vi "Find Endpoint Configuration Section.vi"(8 "error in (no error)":errorcluster, 11 "SLSC Custom Device Ref in":T1 format="%.0x") -> (0 "error out":errorcluster, 2 "Endpoint Config Section Ref":T1 format="%.0x", 3 "SLSC Custom Device  Ref out":T1 format="%.0x")   [LabVIEW 2017, in "SLSC Switch Scripting.lvlib"]
uses:
  SLSC Switch Scripting.lvlib
  <vilib>/NI Veristand/Custom Device API/Custom Device Item Ref.ctl
  NationalInstruments.VeriStand.SystemDefinitionAPI
  SLSC Scripting Constants.vi
  <vilib>/NI VeriStand/Custom Device API/Custom Device API.lvlib
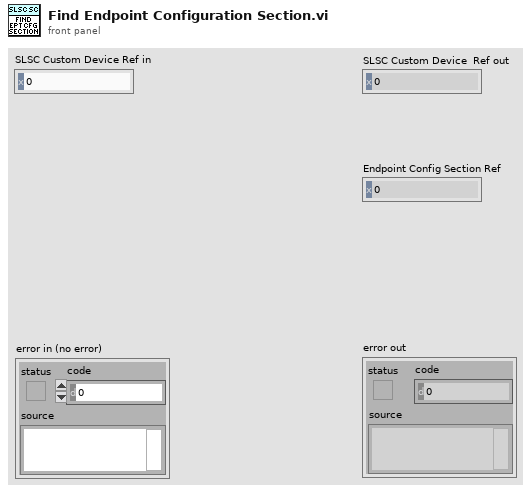
[diagram p1: front panel]
types:
  T1 = typedef "Custom Device API.lvlib/Custom Device Item Ref.ctl" = u64
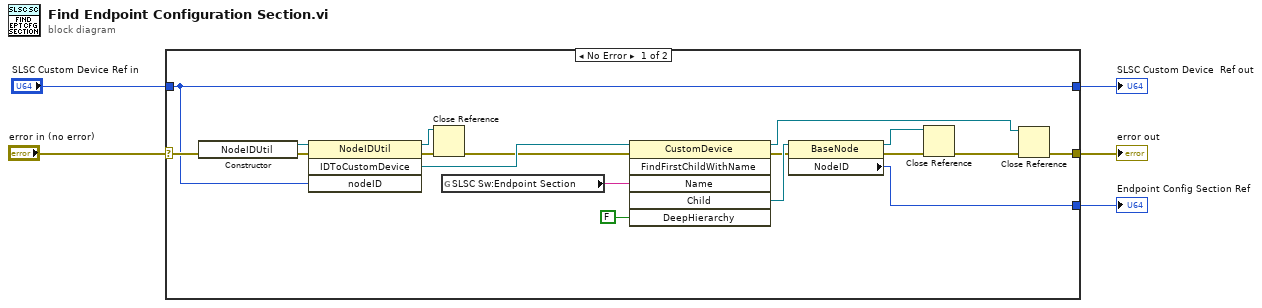
[diagram p0: block diagram]
diagram:
  n1 = case shown="No Error" "error in (no error)" {
    selector: "error in (no error)" -> [w15 w25]
    tunnel: "SLSC Custom Device Ref in" -> [w6 w24]
    tunnel: [w6 w24] -> w4
    tunnel: [w7 w25] -> w3
    tunnel: [w19 _] -> w1
    frame No Error {
      n2 = constructor class="NodeIDUtil"(error in=w15) -> (reference out=w17:refnum<k24>, error out=w18:errorcluster)  [unwired: 2 in, 1 out]
      n3 = invoke class="NodeIDUtil" method="IDToCustomDevice"(reference=w17, error in=w18, "nodeID"=w6) -> (reference out=w13:refnum<k24>, error out=w14:errorcluster, "IDToCustomDevice"=w16:refnum<k24>)  [unwired: 1 in, 1 out]
      n4 = Close Reference(reference=w13, error in (no error)=w14) -> (error out=w12:errorcluster)
      n5 = global read "SLSC Scripting Constants.vi" "SLSC Sw:Endpoint Section"() -> (w23:string)
      n6 = invoke class="CustomDevice" method="FindFirstChildWithName"(reference=w16, error in=w12, "Name"=w23, "DeepHierarchy"=FALSE) -> (reference out=w8:refnum<k24>, error out=w21:errorcluster, "Child"=w22:refnum<k24>)  [unwired: 2 in, 3 out]
      n7 = property class="BaseNode"(reference=w22, error in=w21) -> (reference out=w10:refnum<k24>, error out=w11:errorcluster, "NodeID"=w19:u64)
      n8 = Close Reference(reference=w10, error in (no error)=w11) -> (error out=w9:errorcluster)
      n9 = Close Reference(reference=w8, error in (no error)=w9) -> (error out=w7:errorcluster)
    }
    frame Error {
    }
  }
  "SLSC Custom Device  Ref out" <- w4
  "Endpoint Config Section Ref" <- w1
  "error out" <- w3
